vi "CallBack.vi"(4 "User Parameter":variant, 5 "Event Data":cluster{"sender":refnum<k24>, "e":refnum<k24>}, 6 "Control Ref":refnum<k24>, 7 "Event Common Data":T1) -> ()   [LabVIEW 2017]
uses:
  D:/upwork/Laser Measurement Tool/Laser/tests/KIM101/Thorlabs.MotionControl.KCube.InertialMotorCLI.dll
  Thorlabs.MotionControl.KCube.InertialMotorCLI.dll
panel:
  out "Status":u32
  out "Position":i32
  out "IsMoving":bool
  out "IsError":bool
  out "IsEnabled":bool
  out "Channel":i32(ring)=1 items=["Channel1"=1, "Channel2"=2, "Channel3"=3, "Channel4"=4]
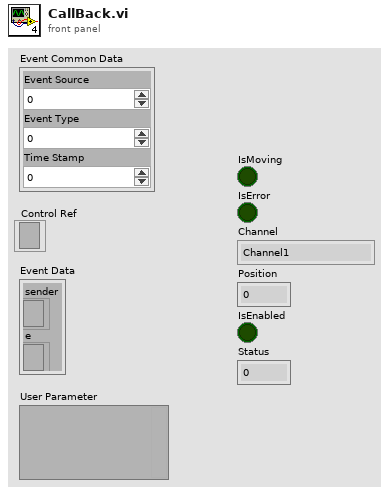
[diagram p1: front panel]
types:
  T1 = cluster{"Event Source":i32, "Event Type":u32, "Time Stamp":u32}
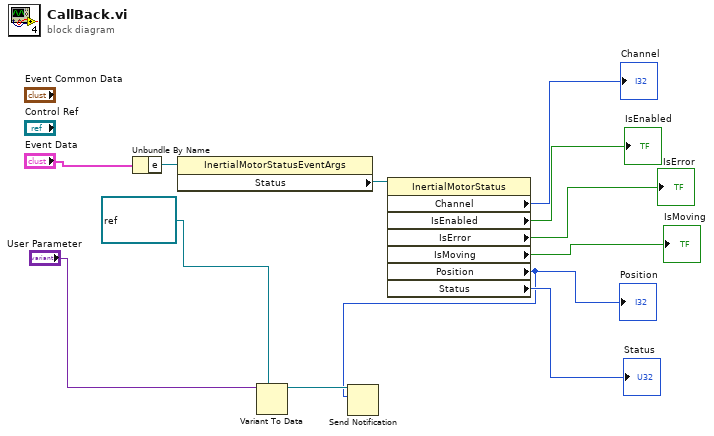
[diagram p0: block diagram]
diagram:
  n1 = Unbundle By Name("Event Data") -> ("e"=w11:refnum<k24>)
  n2 = property class="InertialMotorStatusEventArgs"(reference=w11) -> ("Status"=w10:refnum<k24>)  [unwired: 1 in, 2 out]
  n3 = Variant To Data(type=refnum<notifier> refnum ("notifier out"), Variant="User Parameter") -> (data=w2:refnum<notifier>)  [unwired: 1 in, 1 out]
  n4 = property class="InertialMotorStatus"(reference=w10) -> ("Channel"=→"Channel":i32, "IsEnabled"=→"IsEnabled":bool, "IsError"=→"IsError":bool, "IsMoving"=→"IsMoving":bool, "Position"=w1:i32, "Status"=→"Status":u32)  [unwired: 1 in, 2 out]
  "Position" <- w1
  n5 = Send Notification(notification=w1, notifier=w2) -> ()  [unwired: 1 in, 2 out]
